vi "Toggle Blink.vi"(8 "error in (no error)":errorcluster, 9 "Blinking":bool=TRUE, 10 "Enum":T2(ring), 11 "ROB infocluster ref":T1) -> (0 "error out":errorcluster, 3 "ROB infocluster ref":T1)   [LabVIEW 2016]
uses:
  Typedefs/ROB info refnum.ctl
  Typedefs/ROB display info.ctl
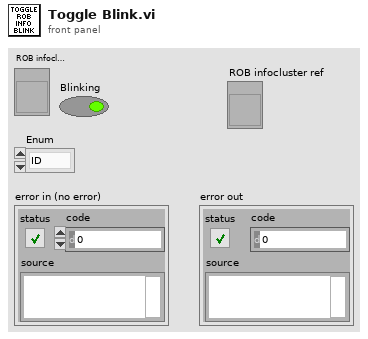
[diagram p1: front panel]
types:
  T1 = typedef "ROB info refnum.ctl" = refnum<vi>
  T2 = enum16{"ID", "Status", "Voltages", "Temp", "Latch count", "VRef", "Trigthres", "MPPC EN?", "Test charge?", "Responding?"}
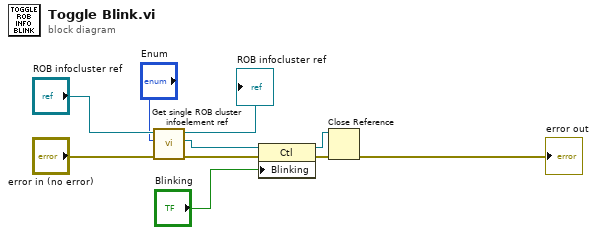
[diagram p0: block diagram]
diagram:
  n1 = call "Get single ROB cluster infoelement ref.vi"("error in (no error)"="error in (no error)", "Enum"="Enum", "ROB infocluster ref"="ROB infocluster ref") -> ("error out"=w2:errorcluster, "Element reference"=w3:refnum<vi>, "ROB infocluster ref"=→"ROB infocluster ref":T1)  [unwired: 6 in]
  n2 = property class="Ctl"(reference=w3, error in=w2, "Blinking"="Blinking") -> (reference out=w9:refnum<vi>, error out=w8:errorcluster)
  n3 = Close Reference(reference=w9, error in (no error)=w8) -> (error out=→"error out":errorcluster)
